vi "Temperature Warnings.vi"(8 "Error In":errorcluster, 11 "Weather Data In":T1={"Current Temperature"=0.0, "Max Temperature"=0.0, "Min Temperature"=0.0, "Warning?"=FALSE, "Warning Text"="No Warning", "Current Windspeed"=0.0, "Max Windspeed"=0.0, "Windspeed Warning?"=FALSE, "Windspeed Warning Text"="No Warning"}) -> (0 "Error Out":errorcluster, 3 "Weather Data Out":T1={"Current Temperature"=0.0, "Max Temperature"=0.0, "Min Temperature"=0.0, "Warning?"=FALSE, "Warning Text"="No Warning", "Current Windspeed"=0.0, "Max Windspeed"=0.0, "Windspeed Warning?"=FALSE, "Windspeed Warning Text"="No Warning"})   [LabVIEW 2022 SP3]
doc: "This VI is used to determine the string to output to the weather station based on the current temperature and limit settings.\n\nInputs: Current Temperature (DBL), Minimum Temperature (DBL), and Maximum Temperature (DBL).\nOutputs: Warning Text (string) and Warning? (Boolean)."
uses:
  Control 1.ctl
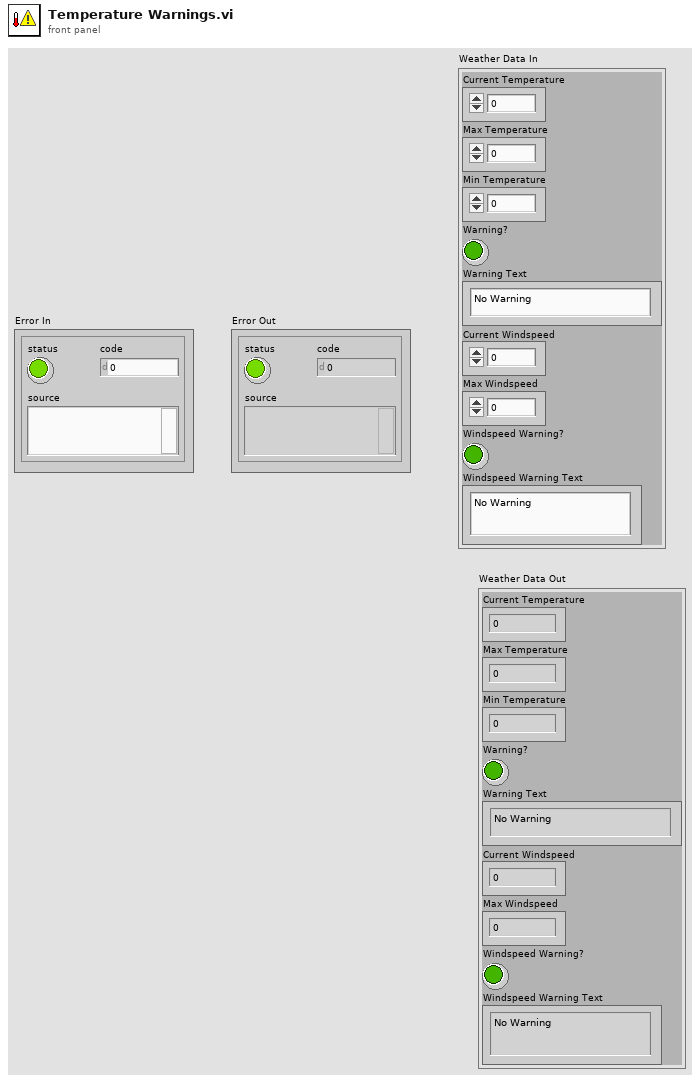
[diagram p1: front panel]
types:
  T1 = typedef "Control 1.ctl" = cluster{"Current Temperature":dbl, "Max Temperature":dbl, "Min Temperature":dbl, "Warning?":bool, "Warning Text":string, "Current Windspeed":dbl, "Max Windspeed":dbl, "Windspeed Warning?":bool, "Windspeed Warning Text":string}
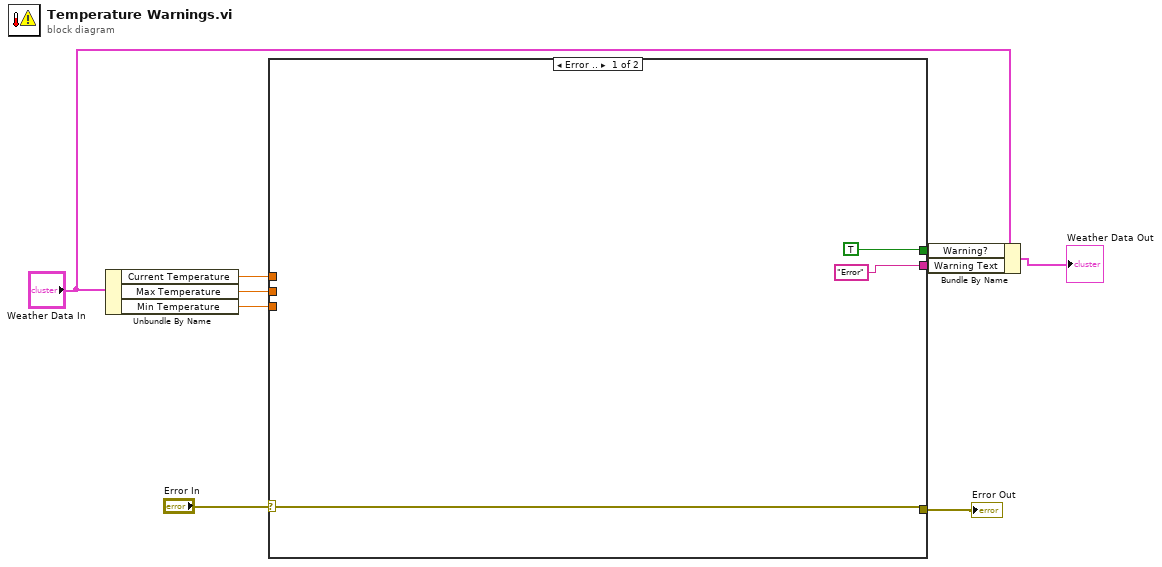
[diagram p0: block diagram]
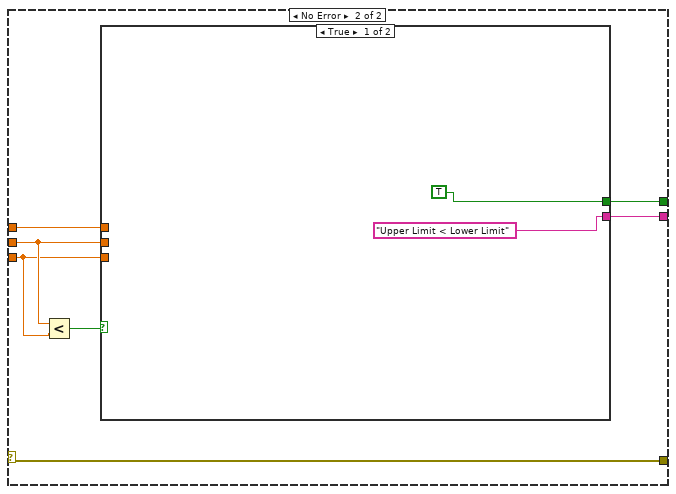
[diagram p2: hidden frame]
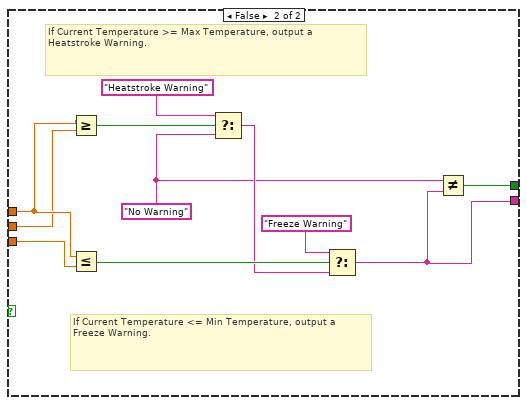
[diagram p3: hidden frame]
diagram:
  n1 = Unbundle By Name("Weather Data In") -> ("Current Temperature"=w5:dbl, "Max Temperature"=w6:dbl, "Min Temperature"=w7:dbl)
  n2 = case shown="Error .." "Error In" {
    selector: "Error In" -> [w12 w13]
    tunnel: [TRUE w19] -> w9
    tunnel: ["Error" w18] -> w8
    tunnel: w7 -> [_ w15]
    tunnel: w6 -> [_ w16]
    tunnel: w5 -> [_ w17]
    tunnel: [w12 w13] -> w1
    frame Error {
    }
    frame No Error {
      n3 = Less?(x=w16, y=w15) -> (x < y?=w14:bool)
      n4 = case shown="True" w14 {
        tunnel: [TRUE w26] -> w19
        tunnel: ["Upper Limit < Lower Limit" w25] -> w18
        tunnel: w17 -> [_ w24]
        tunnel: w16 -> [_ w23]
        tunnel: w15 -> [_ w22]
        frame True {
        }
        frame False {
          w27 = "No Warning" ("f")
          # "If Current Temperature >= Max Temperature, output a Heatstroke Warning."
          # "If Current Temperature <= Min Temperature, output a Freeze Warning."
          n5 = Greater Or Equal?(x=w24, y=w23) -> (x >= y?=w32:bool)
          n6 = Less Or Equal?(x=w24, y=w22) -> (x <= y?=w29:bool)
          n7 = Select(t="Heatstroke Warning", s=w32, f=w27) -> (s? t:f=w28:string)
          n8 = Select(t="Freeze Warning", s=w29, f=w28) -> (s? t:f=w25:string)
          n9 = Not Equal?(x=w27, y=w25) -> (x != y?=w26:bool)
        }
      }
    }
  }
  "Error Out" <- w1
  n10 = Bundle By Name(cluster="Weather Data In", "Warning?"=w9, "Warning Text"=w8) -> (→"Weather Data Out":T1)
